vi "Ytelse.vi"() -> ()   [LabVIEW 2010]
panel:
  out "NextValue 5":sgl(graph)
  out "NextValue 4":sgl
  out "NextValue 3":sgl
  out "NextValue 2":sgl(graph)
  in  "millisecond multiple":u32=1000
  out "Numeric":i32
  out "NextValue":sgl(graph)
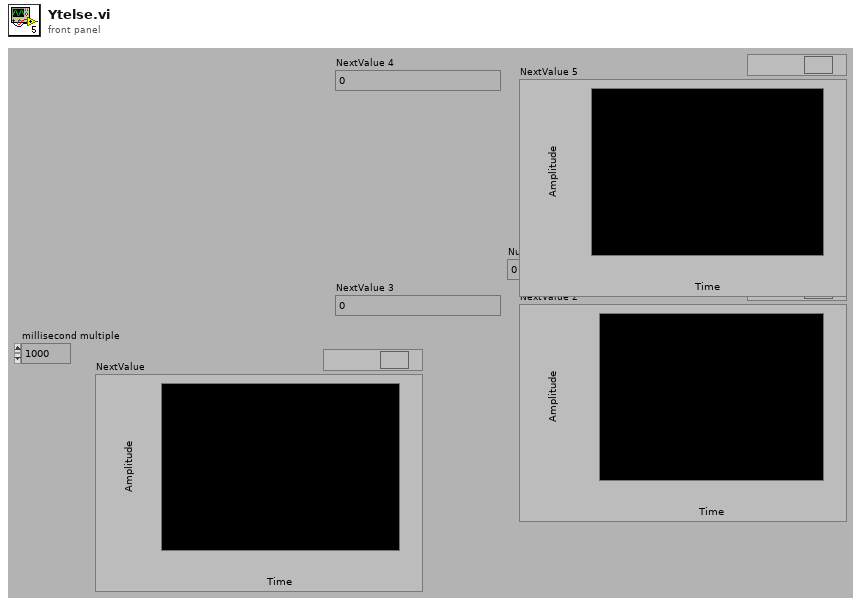
[diagram p1: front panel]
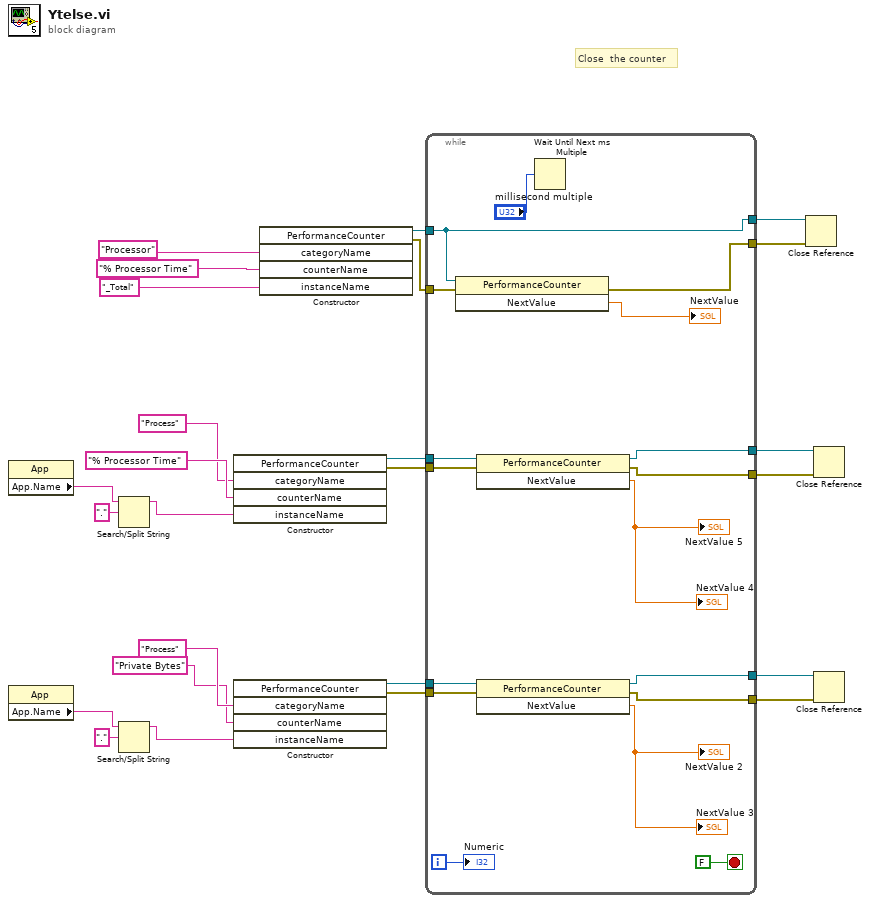
[diagram p0: block diagram]
diagram:
  # "Close  the counter"
  n1 = property class="App"() -> ("App.Name"=w7:string)  [unwired: 2 in, 2 out]
  n2 = property class="App"() -> ("App.Name"=w13:string)  [unwired: 2 in, 2 out]
  n3 = Search/Split String(string=w7, search string/char (-)=".") -> (substring before match=w9:string)  [unwired: 1 in, 2 out]
  n4 = Search/Split String(string=w13, search string/char (-)=".") -> (substring before match=w11:string)  [unwired: 1 in, 2 out]
  n5 = constructor class="PerformanceCounter"("categoryName"="Process", "counterName"="% Processor Time", "instanceName"=w9) -> (reference out=w4:refnum<k24>, error out=w3:errorcluster)  [unwired: 3 in, 4 out]
  n6 = constructor class="PerformanceCounter"("categoryName"="Process", "counterName"="Private Bytes", "instanceName"=w11) -> (reference out=w16:refnum<k24>, error out=w17:errorcluster)  [unwired: 3 in, 4 out]
  n7 = constructor class="PerformanceCounter"("categoryName"="Processor", "counterName"="% Processor Time", "instanceName"="_Total") -> (reference out=w22:refnum<k24>, error out=w20:errorcluster)  [unwired: 3 in, 4 out]
  n8 = while {
    tunnel: w22 -> [w36]
    tunnel: [w36] -> w21
    tunnel: w20 -> [w41]
    tunnel: [w40] -> w19
    tunnel: w17 -> [w35]
    tunnel: w16 -> [w34]
    tunnel: [w33] -> w15
    tunnel: [w32] -> w14
    tunnel: w3 -> [w26]
    tunnel: w4 -> [w27]
    tunnel: [w28] -> w5
    tunnel: [w29] -> w6
    i -> [w38]
    stop <- FALSE stop-if-true
    n9 = invoke class="PerformanceCounter" method="NextValue"(reference=w36, error in=w41) -> (error out=w40:errorcluster, "NextValue"=→"NextValue":sgl)  [unwired: 1 in, 1 out]
    n10 = invoke class="PerformanceCounter" method="NextValue"(reference=w27, error in=w26) -> (reference out=w28:refnum<k24>, error out=w29:errorcluster, "NextValue"=→"NextValue 5" →"NextValue 4":sgl)  [unwired: 1 in]
    n11 = invoke class="PerformanceCounter" method="NextValue"(reference=w34, error in=w35) -> (reference out=w33:refnum<k24>, error out=w32:errorcluster, "NextValue"=→"NextValue 2" →"NextValue 3":sgl)  [unwired: 1 in]
    n12 = Wait Until Next ms Multiple(millisecond multiple="millisecond multiple") -> ()  [unwired: 1 out]
    "Numeric" <- w38
  }
  n13 = Close Reference(reference=w21, error in (no error)=w19) -> ()  [unwired: 1 out]
  n14 = Close Reference(reference=w5, error in (no error)=w6) -> ()  [unwired: 1 out]
  n15 = Close Reference(reference=w15, error in (no error)=w14) -> ()  [unwired: 1 out]
